vi "attributes2Variant.vi"(0 "HGF_PVDataConverter":refnum<class "HGF_PVDataConverter.lvclass">, 2 "Parameter":variant, 3 "typeDescriptor":string, 5 "error in (no error)":errorcluster) -> (14 "HGF_PVDataConverter":refnum<class "HGF_PVDataConverter.lvclass">, 16 "rawData":variant, 19 "error out":errorcluster)   [LabVIEW 2014, in "HGF_BaseClasses.lvlib" / "HGF_PVDataConverter.lvclass"]
doc: "Convert variant attributes Pn, n=0,1,2,... to raw data value of variant."
uses:
  HGF_PVDataConverter.lvclass
  HGF_VariantDataObject/HGF_VariantDataObject.lvclass
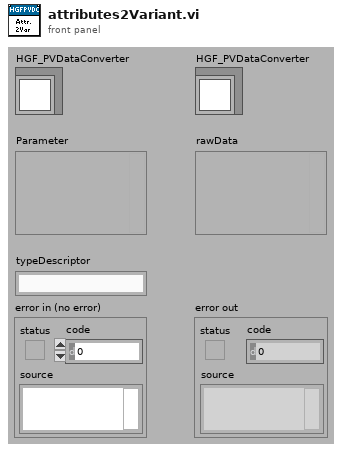
[diagram p1: front panel]
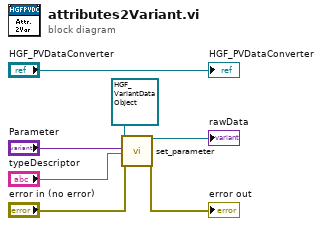
[diagram p0: block diagram]
diagram:
  n1 = call "set_parameter.vi"("HGF_VariantDataObject"=refnum<class "HGF_VariantDataObject.lvclass"> refnum ("HGF_BaseClasses.lvlib:HGF_VariantDataObject.lvclass"), "Parameter"="Parameter", "typeDescriptor"="typeDescriptor", "error in (no error)"="error in (no error)") -> ("dup HGF_VariantDataObject"=→"rawData":refnum<class "HGF_VariantDataObject.lvclass">, "error out"=→"error out":errorcluster)  [unwired: 14 out]
  "HGF_PVDataConverter" <- "HGF_PVDataConverter"
